vi "WILT Step 2.vi"(0 "Dryer Input":T4 {"Night Cycle Count" format="%04d"; "Day Cycle Count" format="%04d"}, 1 "Station Number in":u32, 3 "Send Restart Every? (Sec)":dbl=7.0 format="%#_13g", 5 "Station Test State Cluster":T2, 9 "Current Threshold":dbl=1.0 format="%#_13g", 11 "Error In":errorcluster, 12 "Enable Start Retry":bool, 13 "Delay After Cutout (sec)":dbl, 14 "Agilent Valve and Switch Locations":T1[](array[typedef])) -> (4 "Dryer Output":T4 {"Night Cycle Count" format="%04d"; "Day Cycle Count" format="%04d"}, 6 "Step 2 Output":T2, 10 "Resending Sending Command":bool, 15 "Error Out":errorcluster)   [LabVIEW 2016]
uses:
  Type Definitions/WILT Dryer.ctl
  Type Definitions/WILT Dryer Details.ctl
  Type Definitions/WILT Agilent Channel Definition.ctl
  Type Definitions/WILT DAQ Data.ctl
  Type Definitions/WILT Station Test State Cluster.ctl
  Type Definitions/WILT Dryer Test State.ctl
  Globals/WILT Globals Main Program.vi
panel:
  # "Day"
  # "Night"
  # "Day"
  # "Night"
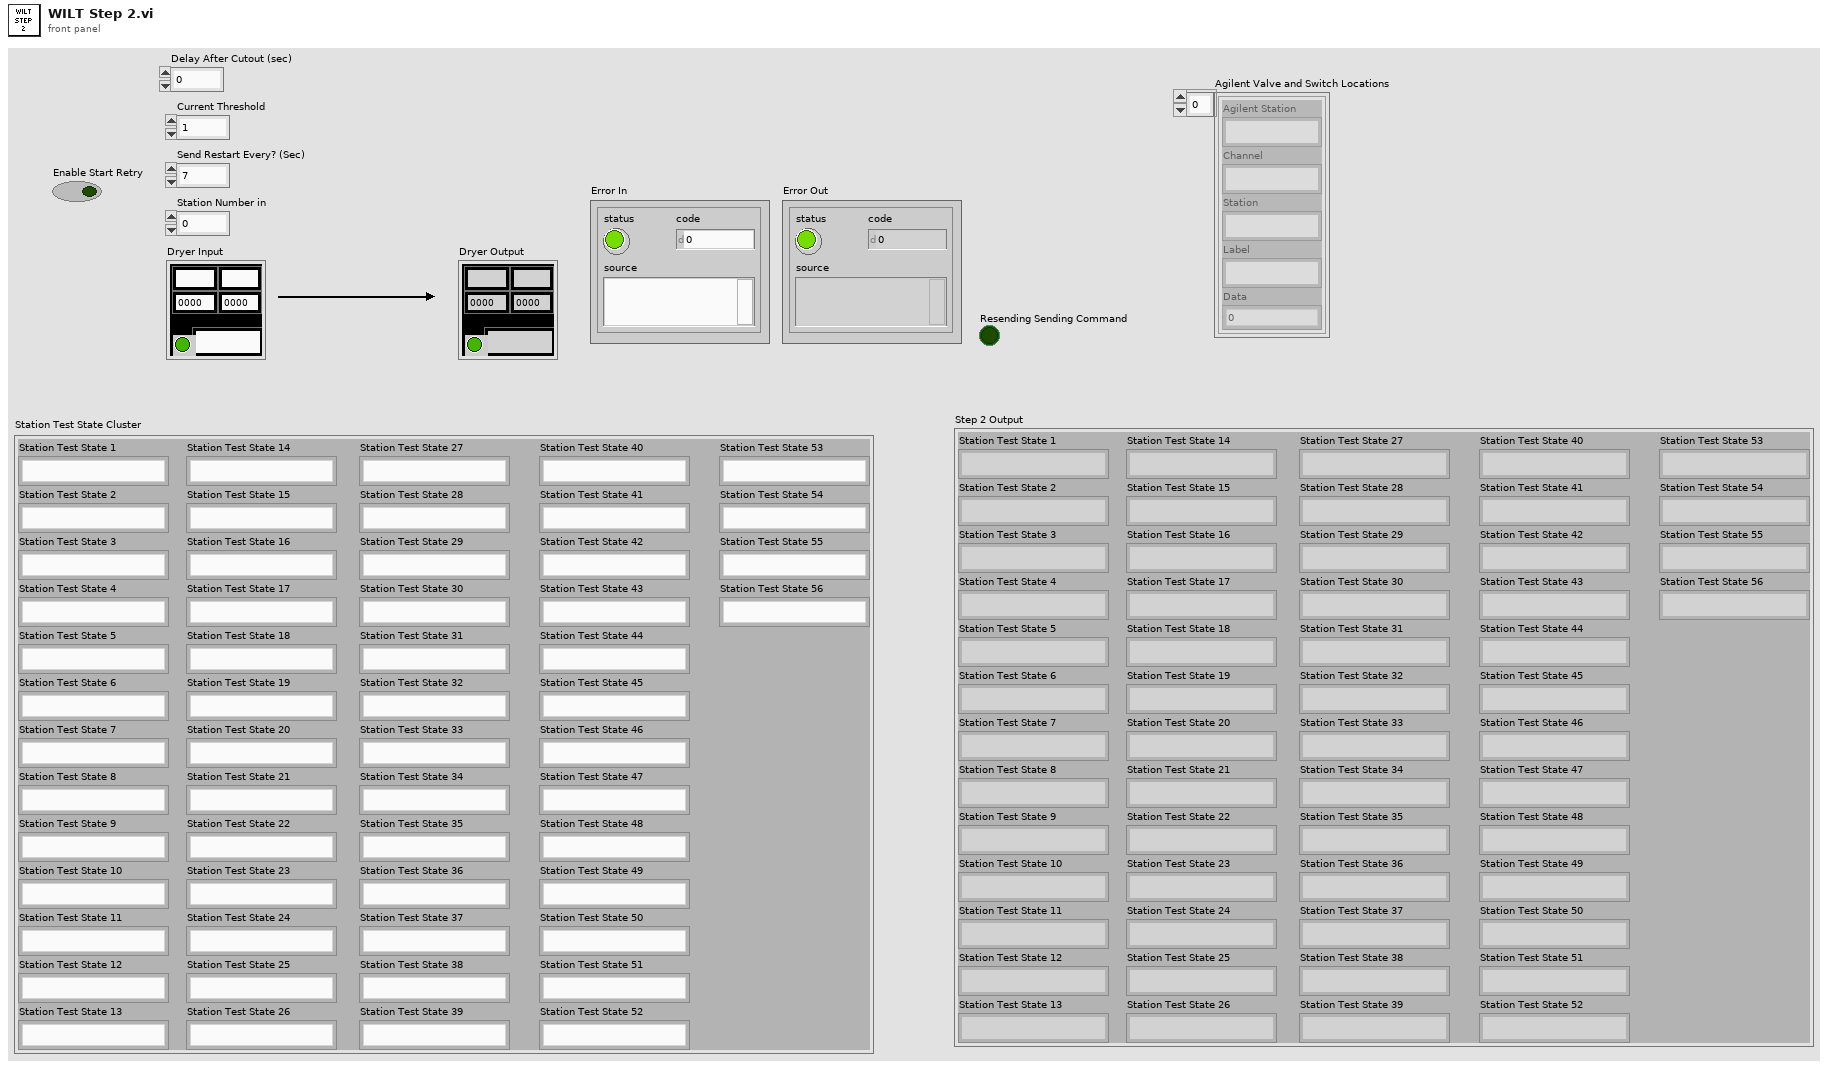
[diagram p1: front panel]
types:
  T1 = typedef "WILT Agilent Channel Definition.ctl" = cluster{"Channel":string, "Station":string, "Label":string, "Agilent Station":string, "Data":dbl}
  T2 = typedef "WILT Station Test State Cluster.ctl" = cluster{"Station Test State 1":T3, "Station Test State 2":T3, "Station Test State 3":T3, "Station Test State 4":T3, "Station Test State 5":T3, "Station Test State 6":T3, "Station Test State 7":T3, "Station Test State 8":T3, "Station Test State 9":T3, "Station Test State 10":T3, "Station Test State 11":T3, "Station Test State 12":T3, "Station Test State 13":T3, "Station Test State 14":T3, "Station Test State 15":T3, "Station Test State 16":T3, "Station Test State 17":T3, "Station Test State 18":T3, "Station Test State 19":T3, "Station Test State 20":T3, "Station Test State 21":T3, "Station Test State 22":T3, "Station Test State 23":T3, "Station Test State 24":T3, "Station Test State 25":T3, "Station Test State 26":T3, "Station Test State 27":T3, "Station Test State 28":T3, "Station Test State 29":T3, "Station Test State 30":T3, "Station Test State 31":T3, "Station Test State 32":T3, "Station Test State 33":T3, "Station Test State 34":T3, "Station Test State 35":T3, "Station Test State 36":T3, "Station Test State 37":T3, "Station Test State 38":T3, "Station Test State 39":T3, "Station Test State 40":T3, "Station Test State 41":T3, "Station Test State 42":T3, "Station Test State 43":T3, "Station Test State 44":T3, "Station Test State 45":T3, "Station Test State 46":T3, "Station Test State 47":T3, "Station Test State 48":T3, "Station Test State 49":T3, "Station Test State 50":T3, "Station Test State 51":T3, "Station Test State 52":T3, "Station Test State 53":T3, "Station Test State 54":T3, "Station Test State 55":T3, "Station Test State 56":T3}
  T3 = typedef "WILT Dryer Test State.ctl" = enum16{"No Serial Number", "Waiting for Dryer To Start", "Drying Clothes", "Water Injection 1 (On)", "Water Injection 1 Timer", "Water Injection 1 (Off)", "Pause Dryer", "Sending Start Stop CMD", "Pause Dryer 2", "Sending Start Stop CMD 2", "Drying Clothes 2", "Water Injection 2 (On)", "Water Injection 2 Timer", "Water Injection 2 (Off)", "Drying Clothes 3", "Cooling Down", "Sending Start Stop CMD 3", "Increment Cycle"}
  T4 = typedef "WILT Dryer.ctl" = cluster{"Lab ID":string, "Day Cycle Count":i32, "Station Label":string, "Dryer Details":T5, "Status Color":u32, "Invisible Button":bool, "Night Cycle Count":i32, "Station Index":i32, "Cycle Index":string, "Audit Alert":bool, "Agilent Channel Definition":T1, "DAQ Data":T6}
  T5 = typedef "WILT Dryer Details.ctl" = cluster{"Station":string, "Lab ID":string, "TR Number":string}
  T6 = typedef "WILT DAQ Data.ctl" = cluster{"L1 Current":dbl, "L2 Current":dbl, "Temperature  Deg F (TC)":dbl, "Volts":dbl, "Volts (208)":dbl, "SW (208)":dbl}
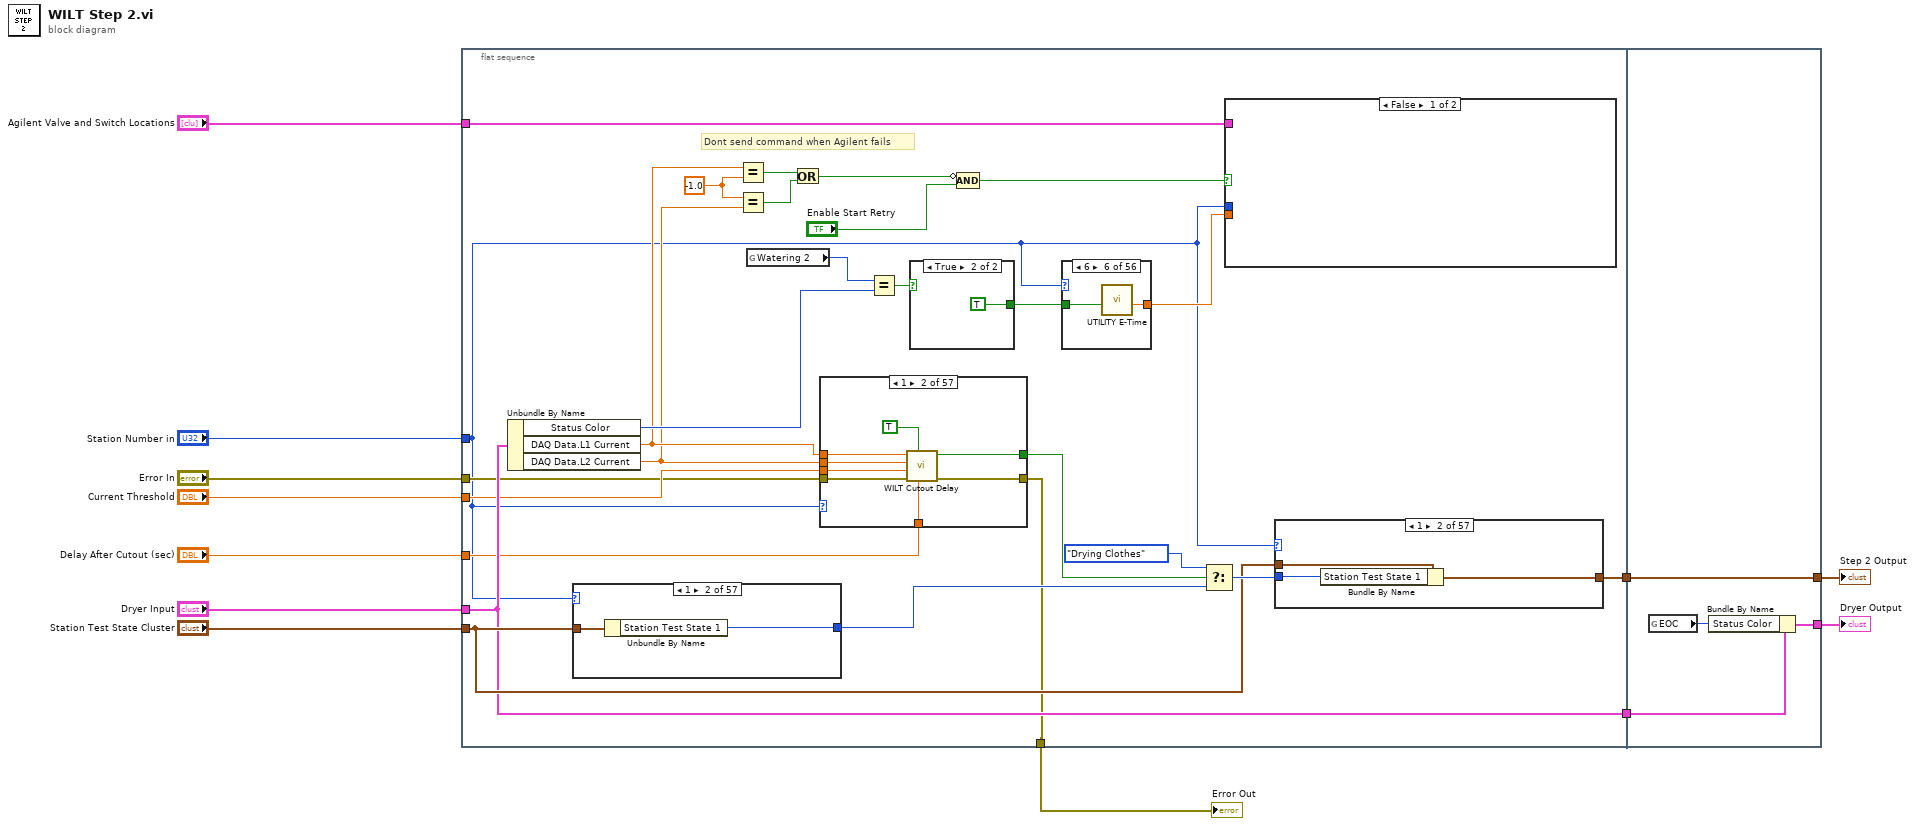
[diagram p0: block diagram]
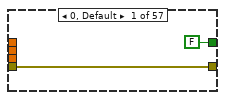
[diagram p2: hidden frame]
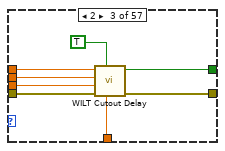
[diagram p3: hidden frame]
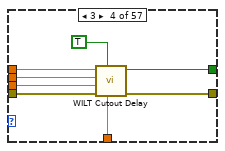
[diagram p4: hidden frame]
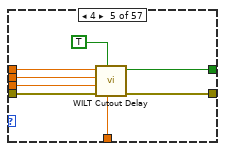
[diagram p5: hidden frame]
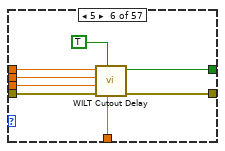
[diagram p6: hidden frame]
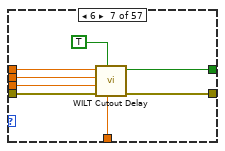
[diagram p7: hidden frame]
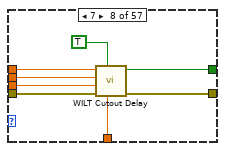
[diagram p8: hidden frame]
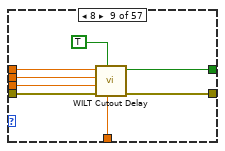
[diagram p9: hidden frame]
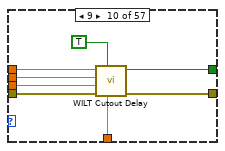
[diagram p10: hidden frame]
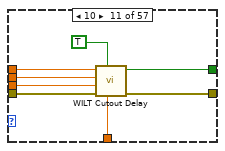
[diagram p11: hidden frame]
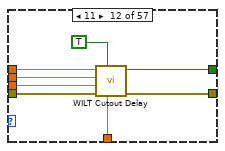
[diagram p12: hidden frame]
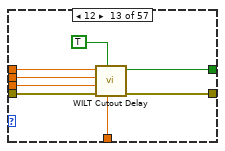
[diagram p13: hidden frame]
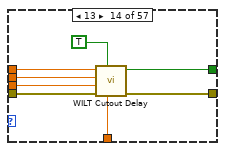
[diagram p14: hidden frame]
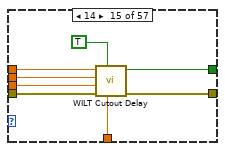
[diagram p15: hidden frame]
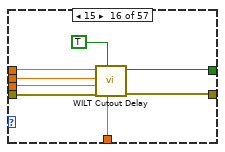
[diagram p16: hidden frame]
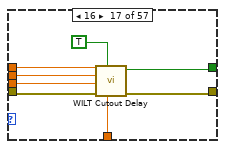
[diagram p17: hidden frame]
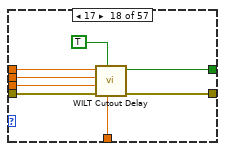
[diagram p18: hidden frame]
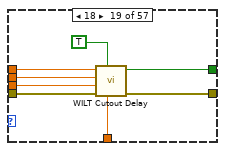
[diagram p19: hidden frame]
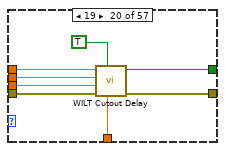
[diagram p20: hidden frame]
diagram:
  n1 = flat-sequence {
    tunnel: "Current Threshold" -> [w18]
    tunnel: "Station Test State Cluster" -> [w35]
    tunnel: "Station Number in" -> [w13]
    tunnel: [w38] -> w8
    tunnel: "Dryer Input" -> [w29]
    tunnel: [w29] -> w6
    tunnel: "Agilent Valve and Switch Locations" -> [w27]
    tunnel: [w16] -> w3
    tunnel: "Error In" -> [w15]
    tunnel: "Delay After Cutout (sec)" -> [w14]
    tunnel: [w893] -> w12
    tunnel: w8 -> [w893]
    tunnel: [w891] -> w7
    tunnel: w6 -> [w890]
    frame #0 {
      w26 = -1.0 ("x")
      # "Dont send command when Agilent fails"
      n2 = Unbundle By Name(w29) -> ("Status Color"=w33:u32, "DAQ Data.L1 Current"=w20:dbl, "DAQ Data.L2 Current"=w19:dbl)
      n3 = case shown="1" w13 {
        tunnel: w35 -> [_ w610 w612 w614 w616 w618 w620 w622 w624 w626 w628 w630 w632 w634 w636 w638 w640 w642 w644 w646 w648 w650 w652 w654 w656 w658 w660 w662 w664 w666 w668 w670 w672 w674 w676 w678 w680 w682 w684 w686 w688 w690 w692 w694 w696 w698 w700 w702 w704 w706 w708 w710 w712 w714 w716 w718 w720]
        tunnel: [WILT_Dryer_Test_State."No Serial Number" ("Station Test State 56") w609 w611 w613 w615 w617 w619 w621 w623 w625 w627 w629 w631 w633 w635 w637 w639 w641 w643 w645 w647 w649 w651 w653 w655 w657 w659 w661 w663 w665 w667 w669 w671 w673 w675 w677 w679 w681 w683 w685 w687 w689 w691 w693 w695 w697 w699 w701 w703 w705 w707 w709 w711 w713 w715 w717 w719] -> w34
        frame 0, Default {
          # "This is not a station.\nDo nothing"
        }
        frame 1 {
          n4 = Unbundle By Name(w610) -> ("Station Test State 1"=w609:T3)
        }
        frame 2 {
          n5 = Unbundle By Name(w612) -> ("Station Test State 2"=w611:T3)
        }
        frame 3 {
          n6 = Unbundle By Name(w614) -> ("Station Test State 3"=w613:T3)
        }
        frame 4 {
          n7 = Unbundle By Name(w616) -> ("Station Test State 4"=w615:T3)
        }
        frame 5 {
          n8 = Unbundle By Name(w618) -> ("Station Test State 5"=w617:T3)
        }
        frame 6 {
          n9 = Unbundle By Name(w620) -> ("Station Test State 6"=w619:T3)
        }
        frame 7 {
          n10 = Unbundle By Name(w622) -> ("Station Test State 7"=w621:T3)
        }
        frame 8 {
          n11 = Unbundle By Name(w624) -> ("Station Test State 8"=w623:T3)
        }
        frame 9 {
          n12 = Unbundle By Name(w626) -> ("Station Test State 9"=w625:T3)
        }
        frame 10 {
          n13 = Unbundle By Name(w628) -> ("Station Test State 10"=w627:T3)
        }
        frame 11 {
          n14 = Unbundle By Name(w630) -> ("Station Test State 11"=w629:T3)
        }
        frame 12 {
          n15 = Unbundle By Name(w632) -> ("Station Test State 12"=w631:T3)
        }
        frame 13 {
          n16 = Unbundle By Name(w634) -> ("Station Test State 13"=w633:T3)
        }
        frame 14 {
          n17 = Unbundle By Name(w636) -> ("Station Test State 14"=w635:T3)
        }
        frame 15 {
          n18 = Unbundle By Name(w638) -> ("Station Test State 15"=w637:T3)
        }
        frame 16 {
          n19 = Unbundle By Name(w640) -> ("Station Test State 16"=w639:T3)
        }
        frame 17 {
          n20 = Unbundle By Name(w642) -> ("Station Test State 17"=w641:T3)
        }
        frame 18 {
          n21 = Unbundle By Name(w644) -> ("Station Test State 18"=w643:T3)
        }
        frame 19 {
          n22 = Unbundle By Name(w646) -> ("Station Test State 19"=w645:T3)
        }
        frame 20 {
          n23 = Unbundle By Name(w648) -> ("Station Test State 20"=w647:T3)
        }
        frame 21 {
          n24 = Unbundle By Name(w650) -> ("Station Test State 21"=w649:T3)
        }
        frame 22 {
          n25 = Unbundle By Name(w652) -> ("Station Test State 22"=w651:T3)
        }
        frame 23 {
          n26 = Unbundle By Name(w654) -> ("Station Test State 23"=w653:T3)
        }
        frame 24 {
          n27 = Unbundle By Name(w656) -> ("Station Test State 24"=w655:T3)
        }
        frame 25 {
          n28 = Unbundle By Name(w658) -> ("Station Test State 25"=w657:T3)
        }
        frame 26 {
          n29 = Unbundle By Name(w660) -> ("Station Test State 26"=w659:T3)
        }
        frame 27 {
          n30 = Unbundle By Name(w662) -> ("Station Test State 27"=w661:T3)
        }
        frame 28 {
          n31 = Unbundle By Name(w664) -> ("Station Test State 28"=w663:T3)
        }
        frame 29 {
          n32 = Unbundle By Name(w666) -> ("Station Test State 29"=w665:T3)
        }
        frame 30 {
          n33 = Unbundle By Name(w668) -> ("Station Test State 30"=w667:T3)
        }
        frame 31 {
          n34 = Unbundle By Name(w670) -> ("Station Test State 31"=w669:T3)
        }
        frame 32 {
          n35 = Unbundle By Name(w672) -> ("Station Test State 32"=w671:T3)
        }
        frame 33 {
          n36 = Unbundle By Name(w674) -> ("Station Test State 33"=w673:T3)
        }
        frame 34 {
          n37 = Unbundle By Name(w676) -> ("Station Test State 34"=w675:T3)
        }
        frame 35 {
          n38 = Unbundle By Name(w678) -> ("Station Test State 35"=w677:T3)
        }
        frame 36 {
          n39 = Unbundle By Name(w680) -> ("Station Test State 36"=w679:T3)
        }
        frame 37 {
          n40 = Unbundle By Name(w682) -> ("Station Test State 37"=w681:T3)
        }
        frame 38 {
          n41 = Unbundle By Name(w684) -> ("Station Test State 38"=w683:T3)
        }
        frame 39 {
          n42 = Unbundle By Name(w686) -> ("Station Test State 39"=w685:T3)
        }
        frame 40 {
          n43 = Unbundle By Name(w688) -> ("Station Test State 40"=w687:T3)
        }
        frame 41 {
          n44 = Unbundle By Name(w690) -> ("Station Test State 41"=w689:T3)
        }
        frame 42 {
          n45 = Unbundle By Name(w692) -> ("Station Test State 42"=w691:T3)
        }
        frame 43 {
          n46 = Unbundle By Name(w694) -> ("Station Test State 43"=w693:T3)
        }
        frame 44 {
          n47 = Unbundle By Name(w696) -> ("Station Test State 44"=w695:T3)
        }
        frame 45 {
          n48 = Unbundle By Name(w698) -> ("Station Test State 45"=w697:T3)
        }
        frame 46 {
          n49 = Unbundle By Name(w700) -> ("Station Test State 46"=w699:T3)
        }
        frame 47 {
          n50 = Unbundle By Name(w702) -> ("Station Test State 47"=w701:T3)
        }
        frame 48 {
          n51 = Unbundle By Name(w704) -> ("Station Test State 48"=w703:T3)
        }
        frame 49 {
          n52 = Unbundle By Name(w706) -> ("Station Test State 49"=w705:T3)
        }
        frame 50 {
          n53 = Unbundle By Name(w708) -> ("Station Test State 50"=w707:T3)
        }
        frame 51 {
          n54 = Unbundle By Name(w710) -> ("Station Test State 51"=w709:T3)
        }
        frame 52 {
          n55 = Unbundle By Name(w712) -> ("Station Test State 52"=w711:T3)
        }
        frame 53 {
          n56 = Unbundle By Name(w714) -> ("Station Test State 53"=w713:T3)
        }
        frame 54 {
          n57 = Unbundle By Name(w716) -> ("Station Test State 54"=w715:T3)
        }
        frame 55 {
          n58 = Unbundle By Name(w718) -> ("Station Test State 55"=w717:T3)
        }
        frame 56 {
          n59 = Unbundle By Name(w720) -> ("Station Test State 56"=w719:T3)
        }
      }
      n60 = Equal?(x=w20, y=w26) -> (x = y?=w25:bool)
      n61 = Equal?(x=w26, y=w19) -> (x = y?=w24:bool)
      n62 = global read "WILT Globals Main Program.vi" "Watering 2"() -> (w32:u32)
      n63 = Or(x=w25, y=w24) -> (x .or. y?=w22:bool)
      n64 = case shown="1" w13 {
        tunnel: w18 -> [_ w48 w51 w59 w70 w78 w86 w94 w102 w110 w118 w126 w134 w142 w150 w155 w166 w174 w182 w190 w198 w206 w214 w222 w230 w238 w246 w254 w262 w270 w278 w286 w294 w302 w310 w318 w326 w334 w342 w350 w358 w366 w374 w382 w390 w398 w406 w414 w422 w430 w438 w446 w454 w462 w470 w478 w486]
        tunnel: w20 -> [_ w47 w53 w61 w72 w80 w88 w96 w104 w112 w120 w128 w136 w144 w152 w157 w168 w176 w184 w192 w200 w208 w216 w224 w232 w240 w248 w256 w264 w272 w280 w288 w296 w304 w312 w320 w328 w336 w344 w352 w360 w368 w376 w384 w392 w400 w408 w416 w424 w432 w440 w448 w456 w464 w472 w480 w488]
        tunnel: w19 -> [_ w46 w52 w60 w71 w79 w87 w95 w103 w111 w119 w127 w135 w143 w151 w156 w167 w175 w183 w191 w199 w207 w215 w223 w231 w239 w247 w255 w263 w271 w279 w287 w295 w303 w311 w319 w327 w335 w343 w351 w359 w367 w375 w383 w391 w399 w407 w415 w423 w431 w439 w447 w455 w463 w471 w479 w487]
        tunnel: [FALSE ("Delayed Trigger") w45 w50 w62 w66 w75 w83 w90 w99 w107 w115 w122 w132 w140 w148 w158 w163 w171 w179 w188 w195 w202 w211 w218 w227 w235 w242 w251 w259 w267 w275 w282 w290 w298 w306 w314 w323 w330 w338 w347 w354 w362 w370 w378 w387 w395 w402 w411 w418 w427 w435 w443 w451 w459 w467 w475 w482] -> w17
        tunnel: w15 -> [w40 w44 w56 w64 w69 w77 w85 w93 w101 w109 w117 w125 w133 w141 w149 w160 w165 w173 w181 w189 w197 w205 w213 w221 w229 w237 w245 w253 w261 w269 w277 w285 w293 w301 w309 w317 w325 w333 w341 w349 w357 w365 w373 w381 w389 w397 w405 w413 w421 w429 w437 w445 w453 w461 w469 w477 w485]
        tunnel: [w40 w43 w55 w63 w67 w76 w82 w91 w100 w108 w114 w123 w131 w139 w147 w159 w164 w172 w180 w187 w196 w203 w210 w219 w228 w234 w243 w252 w260 w268 w276 w283 w291 w299 w307 w315 w324 w331 w339 w348 w355 w363 w371 w379 w388 w396 w403 w412 w419 w428 w436 w444 w452 w460 w468 w476 w483] -> w16
        tunnel: w14 -> [_ w42 w54 w58 w68 w74 w84 w92 w98 w106 w116 w124 w130 w138 w146 w154 w162 w170 w178 w186 w194 w204 w212 w220 w226 w236 w244 w250 w258 w266 w274 w284 w292 w300 w308 w316 w322 w332 w340 w346 w356 w364 w372 w380 w386 w394 w404 w410 w420 w426 w434 w442 w450 w458 w466 w474 w484]
        frame 0, Default {
        }
        frame 1 {
          n65 = call "WILT Cutout Delay.vi"("Delay After Cutout (sec)"=w42, "Cut-In?"=TRUE, "Error In"=w44, "Current Threshold"=w48, "L2 Current"=w46, "L1 Current"=w47) -> ("Error Out"=w43:errorcluster, "Delayed Trigger"=w45:bool)  [unwired: 2 in, 2 out]
        }
        frame 2 {
          n66 = call "WILT Cutout Delay.vi"("Delay After Cutout (sec)"=w54, "Cut-In?"=TRUE, "Error In"=w56, "Current Threshold"=w51, "L2 Current"=w52, "L1 Current"=w53) -> ("Error Out"=w55:errorcluster, "Delayed Trigger"=w50:bool)  [unwired: 2 in, 2 out]
        }
        frame 3 {
          n67 = call "WILT Cutout Delay.vi"("Delay After Cutout (sec)"=w58, "Cut-In?"=TRUE, "Error In"=w64, "Current Threshold"=w59, "L2 Current"=w60, "L1 Current"=w61) -> ("Error Out"=w63:errorcluster, "Delayed Trigger"=w62:bool)  [unwired: 2 in, 2 out]
        }
        frame 4 {
          n68 = call "WILT Cutout Delay.vi"("Delay After Cutout (sec)"=w68, "Cut-In?"=TRUE, "Error In"=w69, "Current Threshold"=w70, "L2 Current"=w71, "L1 Current"=w72) -> ("Error Out"=w67:errorcluster, "Delayed Trigger"=w66:bool)  [unwired: 2 in, 2 out]
        }
        frame 5 {
          n69 = call "WILT Cutout Delay.vi"("Delay After Cutout (sec)"=w74, "Cut-In?"=TRUE, "Error In"=w77, "Current Threshold"=w78, "L2 Current"=w79, "L1 Current"=w80) -> ("Error Out"=w76:errorcluster, "Delayed Trigger"=w75:bool)  [unwired: 2 in, 2 out]
        }
        frame 6 {
          n70 = call "WILT Cutout Delay.vi"("Delay After Cutout (sec)"=w84, "Cut-In?"=TRUE, "Error In"=w85, "Current Threshold"=w86, "L2 Current"=w87, "L1 Current"=w88) -> ("Error Out"=w82:errorcluster, "Delayed Trigger"=w83:bool)  [unwired: 2 in, 2 out]
        }
        frame 7 {
          n71 = call "WILT Cutout Delay.vi"("Delay After Cutout (sec)"=w92, "Cut-In?"=TRUE, "Error In"=w93, "Current Threshold"=w94, "L2 Current"=w95, "L1 Current"=w96) -> ("Error Out"=w91:errorcluster, "Delayed Trigger"=w90:bool)  [unwired: 2 in, 2 out]
        }
        frame 8 {
          n72 = call "WILT Cutout Delay.vi"("Delay After Cutout (sec)"=w98, "Cut-In?"=TRUE, "Error In"=w101, "Current Threshold"=w102, "L2 Current"=w103, "L1 Current"=w104) -> ("Error Out"=w100:errorcluster, "Delayed Trigger"=w99:bool)  [unwired: 2 in, 2 out]
        }
        frame 9 {
          n73 = call "WILT Cutout Delay.vi"("Delay After Cutout (sec)"=w106, "Cut-In?"=TRUE, "Error In"=w109, "Current Threshold"=w110, "L2 Current"=w111, "L1 Current"=w112) -> ("Error Out"=w108:errorcluster, "Delayed Trigger"=w107:bool)  [unwired: 2 in, 2 out]
        }
        frame 10 {
          n74 = call "WILT Cutout Delay.vi"("Delay After Cutout (sec)"=w116, "Cut-In?"=TRUE, "Error In"=w117, "Current Threshold"=w118, "L2 Current"=w119, "L1 Current"=w120) -> ("Error Out"=w114:errorcluster, "Delayed Trigger"=w115:bool)  [unwired: 2 in, 2 out]
        }
        frame 11 {
          n75 = call "WILT Cutout Delay.vi"("Delay After Cutout (sec)"=w124, "Cut-In?"=TRUE, "Error In"=w125, "Current Threshold"=w126, "L2 Current"=w127, "L1 Current"=w128) -> ("Error Out"=w123:errorcluster, "Delayed Trigger"=w122:bool)  [unwired: 2 in, 2 out]
        }
        frame 12 {
          n76 = call "WILT Cutout Delay.vi"("Delay After Cutout (sec)"=w130, "Cut-In?"=TRUE, "Error In"=w133, "Current Threshold"=w134, "L2 Current"=w135, "L1 Current"=w136) -> ("Error Out"=w131:errorcluster, "Delayed Trigger"=w132:bool)  [unwired: 2 in, 2 out]
        }
        frame 13 {
          n77 = call "WILT Cutout Delay.vi"("Delay After Cutout (sec)"=w138, "Cut-In?"=TRUE, "Error In"=w141, "Current Threshold"=w142, "L2 Current"=w143, "L1 Current"=w144) -> ("Error Out"=w139:errorcluster, "Delayed Trigger"=w140:bool)  [unwired: 2 in, 2 out]
        }
        frame 14 {
          n78 = call "WILT Cutout Delay.vi"("Delay After Cutout (sec)"=w146, "Cut-In?"=TRUE, "Error In"=w149, "Current Threshold"=w150, "L2 Current"=w151, "L1 Current"=w152) -> ("Error Out"=w147:errorcluster, "Delayed Trigger"=w148:bool)  [unwired: 2 in, 2 out]
        }
        frame 15 {
          n79 = call "WILT Cutout Delay.vi"("Delay After Cutout (sec)"=w154, "Cut-In?"=TRUE, "Error In"=w160, "Current Threshold"=w155, "L2 Current"=w156, "L1 Current"=w157) -> ("Error Out"=w159:errorcluster, "Delayed Trigger"=w158:bool)  [unwired: 2 in, 2 out]
        }
        frame 16 {
          n80 = call "WILT Cutout Delay.vi"("Delay After Cutout (sec)"=w162, "Cut-In?"=TRUE, "Error In"=w165, "Current Threshold"=w166, "L2 Current"=w167, "L1 Current"=w168) -> ("Error Out"=w164:errorcluster, "Delayed Trigger"=w163:bool)  [unwired: 2 in, 2 out]
        }
        frame 17 {
          n81 = call "WILT Cutout Delay.vi"("Delay After Cutout (sec)"=w170, "Cut-In?"=TRUE, "Error In"=w173, "Current Threshold"=w174, "L2 Current"=w175, "L1 Current"=w176) -> ("Error Out"=w172:errorcluster, "Delayed Trigger"=w171:bool)  [unwired: 2 in, 2 out]
        }
        frame 18 {
          n82 = call "WILT Cutout Delay.vi"("Delay After Cutout (sec)"=w178, "Cut-In?"=TRUE, "Error In"=w181, "Current Threshold"=w182, "L2 Current"=w183, "L1 Current"=w184) -> ("Error Out"=w180:errorcluster, "Delayed Trigger"=w179:bool)  [unwired: 2 in, 2 out]
        }
        frame 19 {
          n83 = call "WILT Cutout Delay.vi"("Delay After Cutout (sec)"=w186, "Cut-In?"=TRUE, "Error In"=w189, "Current Threshold"=w190, "L2 Current"=w191, "L1 Current"=w192) -> ("Error Out"=w187:errorcluster, "Delayed Trigger"=w188:bool)  [unwired: 2 in, 2 out]
        }
        frame 20 {
          n84 = call "WILT Cutout Delay.vi"("Delay After Cutout (sec)"=w194, "Cut-In?"=TRUE, "Error In"=w197, "Current Threshold"=w198, "L2 Current"=w199, "L1 Current"=w200) -> ("Error Out"=w196:errorcluster, "Delayed Trigger"=w195:bool)  [unwired: 2 in, 2 out]
        }
        frame 21 {
          n85 = call "WILT Cutout Delay.vi"("Delay After Cutout (sec)"=w204, "Cut-In?"=TRUE, "Error In"=w205, "Current Threshold"=w206, "L2 Current"=w207, "L1 Current"=w208) -> ("Error Out"=w203:errorcluster, "Delayed Trigger"=w202:bool)  [unwired: 2 in, 2 out]
        }
        frame 22 {
          n86 = call "WILT Cutout Delay.vi"("Delay After Cutout (sec)"=w212, "Cut-In?"=TRUE, "Error In"=w213, "Current Threshold"=w214, "L2 Current"=w215, "L1 Current"=w216) -> ("Error Out"=w210:errorcluster, "Delayed Trigger"=w211:bool)  [unwired: 2 in, 2 out]
        }
        frame 23 {
          n87 = call "WILT Cutout Delay.vi"("Delay After Cutout (sec)"=w220, "Cut-In?"=TRUE, "Error In"=w221, "Current Threshold"=w222, "L2 Current"=w223, "L1 Current"=w224) -> ("Error Out"=w219:errorcluster, "Delayed Trigger"=w218:bool)  [unwired: 2 in, 2 out]
        }
        frame 24 {
          n88 = call "WILT Cutout Delay.vi"("Delay After Cutout (sec)"=w226, "Cut-In?"=TRUE, "Error In"=w229, "Current Threshold"=w230, "L2 Current"=w231, "L1 Current"=w232) -> ("Error Out"=w228:errorcluster, "Delayed Trigger"=w227:bool)  [unwired: 2 in, 2 out]
        }
        frame 25 {
          n89 = call "WILT Cutout Delay.vi"("Delay After Cutout (sec)"=w236, "Cut-In?"=TRUE, "Error In"=w237, "Current Threshold"=w238, "L2 Current"=w239, "L1 Current"=w240) -> ("Error Out"=w234:errorcluster, "Delayed Trigger"=w235:bool)  [unwired: 2 in, 2 out]
        }
        frame 26 {
          n90 = call "WILT Cutout Delay.vi"("Delay After Cutout (sec)"=w244, "Cut-In?"=TRUE, "Error In"=w245, "Current Threshold"=w246, "L2 Current"=w247, "L1 Current"=w248) -> ("Error Out"=w243:errorcluster, "Delayed Trigger"=w242:bool)  [unwired: 2 in, 2 out]
        }
        frame 27 {
          n91 = call "WILT Cutout Delay.vi"("Delay After Cutout (sec)"=w250, "Cut-In?"=TRUE, "Error In"=w253, "Current Threshold"=w254, "L2 Current"=w255, "L1 Current"=w256) -> ("Error Out"=w252:errorcluster, "Delayed Trigger"=w251:bool)  [unwired: 2 in, 2 out]
        }
        frame 28 {
          n92 = call "WILT Cutout Delay.vi"("Delay After Cutout (sec)"=w258, "Cut-In?"=TRUE, "Error In"=w261, "Current Threshold"=w262, "L2 Current"=w263, "L1 Current"=w264) -> ("Error Out"=w260:errorcluster, "Delayed Trigger"=w259:bool)  [unwired: 2 in, 2 out]
        }
        frame 29 {
          n93 = call "WILT Cutout Delay.vi"("Delay After Cutout (sec)"=w266, "Cut-In?"=TRUE, "Error In"=w269, "Current Threshold"=w270, "L2 Current"=w271, "L1 Current"=w272) -> ("Error Out"=w268:errorcluster, "Delayed Trigger"=w267:bool)  [unwired: 2 in, 2 out]
        }
        frame 30 {
          n94 = call "WILT Cutout Delay.vi"("Delay After Cutout (sec)"=w274, "Cut-In?"=TRUE, "Error In"=w277, "Current Threshold"=w278, "L2 Current"=w279, "L1 Current"=w280) -> ("Error Out"=w276:errorcluster, "Delayed Trigger"=w275:bool)  [unwired: 2 in, 2 out]
        }
        frame 31 {
          n95 = call "WILT Cutout Delay.vi"("Delay After Cutout (sec)"=w284, "Cut-In?"=TRUE, "Error In"=w285, "Current Threshold"=w286, "L2 Current"=w287, "L1 Current"=w288) -> ("Error Out"=w283:errorcluster, "Delayed Trigger"=w282:bool)  [unwired: 2 in, 2 out]
        }
        frame 32 {
          n96 = call "WILT Cutout Delay.vi"("Delay After Cutout (sec)"=w292, "Cut-In?"=TRUE, "Error In"=w293, "Current Threshold"=w294, "L2 Current"=w295, "L1 Current"=w296) -> ("Error Out"=w291:errorcluster, "Delayed Trigger"=w290:bool)  [unwired: 2 in, 2 out]
        }
        frame 33 {
          n97 = call "WILT Cutout Delay.vi"("Delay After Cutout (sec)"=w300, "Cut-In?"=TRUE, "Error In"=w301, "Current Threshold"=w302, "L2 Current"=w303, "L1 Current"=w304) -> ("Error Out"=w299:errorcluster, "Delayed Trigger"=w298:bool)  [unwired: 2 in, 2 out]
        }
        frame 34 {
          n98 = call "WILT Cutout Delay.vi"("Delay After Cutout (sec)"=w308, "Cut-In?"=TRUE, "Error In"=w309, "Current Threshold"=w310, "L2 Current"=w311, "L1 Current"=w312) -> ("Error Out"=w307:errorcluster, "Delayed Trigger"=w306:bool)  [unwired: 2 in, 2 out]
        }
        frame 35 {
          n99 = call "WILT Cutout Delay.vi"("Delay After Cutout (sec)"=w316, "Cut-In?"=TRUE, "Error In"=w317, "Current Threshold"=w318, "L2 Current"=w319, "L1 Current"=w320) -> ("Error Out"=w315:errorcluster, "Delayed Trigger"=w314:bool)  [unwired: 2 in, 2 out]
        }
        frame 36 {
          n100 = call "WILT Cutout Delay.vi"("Delay After Cutout (sec)"=w322, "Cut-In?"=TRUE, "Error In"=w325, "Current Threshold"=w326, "L2 Current"=w327, "L1 Current"=w328) -> ("Error Out"=w324:errorcluster, "Delayed Trigger"=w323:bool)  [unwired: 2 in, 2 out]
        }
        frame 37 {
          n101 = call "WILT Cutout Delay.vi"("Delay After Cutout (sec)"=w332, "Cut-In?"=TRUE, "Error In"=w333, "Current Threshold"=w334, "L2 Current"=w335, "L1 Current"=w336) -> ("Error Out"=w331:errorcluster, "Delayed Trigger"=w330:bool)  [unwired: 2 in, 2 out]
        }
        frame 38 {
          n102 = call "WILT Cutout Delay.vi"("Delay After Cutout (sec)"=w340, "Cut-In?"=TRUE, "Error In"=w341, "Current Threshold"=w342, "L2 Current"=w343, "L1 Current"=w344) -> ("Error Out"=w339:errorcluster, "Delayed Trigger"=w338:bool)  [unwired: 2 in, 2 out]
        }
        frame 39 {
          n103 = call "WILT Cutout Delay.vi"("Delay After Cutout (sec)"=w346, "Cut-In?"=TRUE, "Error In"=w349, "Current Threshold"=w350, "L2 Current"=w351, "L1 Current"=w352) -> ("Error Out"=w348:errorcluster, "Delayed Trigger"=w347:bool)  [unwired: 2 in, 2 out]
        }
        frame 40 {
          n104 = call "WILT Cutout Delay.vi"("Delay After Cutout (sec)"=w356, "Cut-In?"=TRUE, "Error In"=w357, "Current Threshold"=w358, "L2 Current"=w359, "L1 Current"=w360) -> ("Error Out"=w355:errorcluster, "Delayed Trigger"=w354:bool)  [unwired: 2 in, 2 out]
        }
        frame 41 {
          n105 = call "WILT Cutout Delay.vi"("Delay After Cutout (sec)"=w364, "Cut-In?"=TRUE, "Error In"=w365, "Current Threshold"=w366, "L2 Current"=w367, "L1 Current"=w368) -> ("Error Out"=w363:errorcluster, "Delayed Trigger"=w362:bool)  [unwired: 2 in, 2 out]
        }
        frame 42 {
          n106 = call "WILT Cutout Delay.vi"("Delay After Cutout (sec)"=w372, "Cut-In?"=TRUE, "Error In"=w373, "Current Threshold"=w374, "L2 Current"=w375, "L1 Current"=w376) -> ("Error Out"=w371:errorcluster, "Delayed Trigger"=w370:bool)  [unwired: 2 in, 2 out]
        }
        frame 43 {
          n107 = call "WILT Cutout Delay.vi"("Delay After Cutout (sec)"=w380, "Cut-In?"=TRUE, "Error In"=w381, "Current Threshold"=w382, "L2 Current"=w383, "L1 Current"=w384) -> ("Error Out"=w379:errorcluster, "Delayed Trigger"=w378:bool)  [unwired: 2 in, 2 out]
        }
        frame 44 {
          n108 = call "WILT Cutout Delay.vi"("Delay After Cutout (sec)"=w386, "Cut-In?"=TRUE, "Error In"=w389, "Current Threshold"=w390, "L2 Current"=w391, "L1 Current"=w392) -> ("Error Out"=w388:errorcluster, "Delayed Trigger"=w387:bool)  [unwired: 2 in, 2 out]
        }
        frame 45 {
          n109 = call "WILT Cutout Delay.vi"("Delay After Cutout (sec)"=w394, "Cut-In?"=TRUE, "Error In"=w397, "Current Threshold"=w398, "L2 Current"=w399, "L1 Current"=w400) -> ("Error Out"=w396:errorcluster, "Delayed Trigger"=w395:bool)  [unwired: 2 in, 2 out]
        }
        frame 46 {
          n110 = call "WILT Cutout Delay.vi"("Delay After Cutout (sec)"=w404, "Cut-In?"=TRUE, "Error In"=w405, "Current Threshold"=w406, "L2 Current"=w407, "L1 Current"=w408) -> ("Error Out"=w403:errorcluster, "Delayed Trigger"=w402:bool)  [unwired: 2 in, 2 out]
        }
        frame 47 {
          n111 = call "WILT Cutout Delay.vi"("Delay After Cutout (sec)"=w410, "Cut-In?"=TRUE, "Error In"=w413, "Current Threshold"=w414, "L2 Current"=w415, "L1 Current"=w416) -> ("Error Out"=w412:errorcluster, "Delayed Trigger"=w411:bool)  [unwired: 2 in, 2 out]
        }
        frame 48 {
          n112 = call "WILT Cutout Delay.vi"("Delay After Cutout (sec)"=w420, "Cut-In?"=TRUE, "Error In"=w421, "Current Threshold"=w422, "L2 Current"=w423, "L1 Current"=w424) -> ("Error Out"=w419:errorcluster, "Delayed Trigger"=w418:bool)  [unwired: 2 in, 2 out]
        }
        frame 49 {
          n113 = call "WILT Cutout Delay.vi"("Delay After Cutout (sec)"=w426, "Cut-In?"=TRUE, "Error In"=w429, "Current Threshold"=w430, "L2 Current"=w431, "L1 Current"=w432) -> ("Error Out"=w428:errorcluster, "Delayed Trigger"=w427:bool)  [unwired: 2 in, 2 out]
        }
        frame 50 {
          n114 = call "WILT Cutout Delay.vi"("Delay After Cutout (sec)"=w434, "Cut-In?"=TRUE, "Error In"=w437, "Current Threshold"=w438, "L2 Current"=w439, "L1 Current"=w440) -> ("Error Out"=w436:errorcluster, "Delayed Trigger"=w435:bool)  [unwired: 2 in, 2 out]
        }
        frame 51 {
          n115 = call "WILT Cutout Delay.vi"("Delay After Cutout (sec)"=w442, "Cut-In?"=TRUE, "Error In"=w445, "Current Threshold"=w446, "L2 Current"=w447, "L1 Current"=w448) -> ("Error Out"=w444:errorcluster, "Delayed Trigger"=w443:bool)  [unwired: 2 in, 2 out]
        }
        frame 52 {
          n116 = call "WILT Cutout Delay.vi"("Delay After Cutout (sec)"=w450, "Cut-In?"=TRUE, "Error In"=w453, "Current Threshold"=w454, "L2 Current"=w455, "L1 Current"=w456) -> ("Error Out"=w452:errorcluster, "Delayed Trigger"=w451:bool)  [unwired: 2 in, 2 out]
        }
        frame 53 {
          n117 = call "WILT Cutout Delay.vi"("Delay After Cutout (sec)"=w458, "Cut-In?"=TRUE, "Error In"=w461, "Current Threshold"=w462, "L2 Current"=w463, "L1 Current"=w464) -> ("Error Out"=w460:errorcluster, "Delayed Trigger"=w459:bool)  [unwired: 2 in, 2 out]
        }
        frame 54 {
          n118 = call "WILT Cutout Delay.vi"("Delay After Cutout (sec)"=w466, "Cut-In?"=TRUE, "Error In"=w469, "Current Threshold"=w470, "L2 Current"=w471, "L1 Current"=w472) -> ("Error Out"=w468:errorcluster, "Delayed Trigger"=w467:bool)  [unwired: 2 in, 2 out]
        }
        frame 55 {
          n119 = call "WILT Cutout Delay.vi"("Delay After Cutout (sec)"=w474, "Cut-In?"=TRUE, "Error In"=w477, "Current Threshold"=w478, "L2 Current"=w479, "L1 Current"=w480) -> ("Error Out"=w476:errorcluster, "Delayed Trigger"=w475:bool)  [unwired: 2 in, 2 out]
        }
        frame 56 {
          n120 = call "WILT Cutout Delay.vi"("Delay After Cutout (sec)"=w484, "Cut-In?"=TRUE, "Error In"=w485, "Current Threshold"=w486, "L2 Current"=w487, "L1 Current"=w488) -> ("Error Out"=w483:errorcluster, "Delayed Trigger"=w482:bool)  [unwired: 2 in, 2 out]
        }
      }
      n121 = Equal?(x=w32, y=w33) -> (x = y?=w31:bool)
      n122 = case shown="True" w31 {
        tunnel: [FALSE TRUE] -> w30
        frame False {
        }
        frame True {
        }
      }
      n123 = Compound Arithmetic op=AND(invert w22, "Enable Start Retry") -> (w21:bool)
      n124 = case shown="6" w13 {
        tunnel: [w497 w498 w500 w502 w504 w506 w508 w510 w512 w514 w516 w518 w520 w522 w524 w526 w528 w530 w532 w534 w536 w538 w540 w542 w544 w546 w548 w550 w552 w554 w556 w558 w560 w562 w564 w566 w568 w570 w572 w574 w576 w578 w580 w582 w584 w586 w588 w590 w592 w594 w596 w598 w600 w602 w604 w606] -> w28
        tunnel: w30 -> [w496 w499 w501 w503 w505 w507 w509 w511 w513 w515 w517 w519 w521 w523 w525 w527 w529 w531 w533 w535 w537 w539 w541 w543 w545 w547 w549 w551 w553 w555 w557 w559 w561 w563 w565 w567 w569 w571 w573 w575 w577 w579 w581 w583 w585 w587 w589 w591 w593 w595 w597 w599 w601 w603 w605 w607]
        frame 1, Default {
          n125 = call "UTILITY E-Time.vi"("Reset"=w496) -> ("Elapsed Time (sec)"=w497:dbl)  [unwired: 8 in, 2 out]
        }
        frame 2 {
          n126 = call "UTILITY E-Time.vi"("Reset"=w499) -> ("Elapsed Time (sec)"=w498:dbl)  [unwired: 8 in, 2 out]
        }
        frame 3 {
          n127 = call "UTILITY E-Time.vi"("Reset"=w501) -> ("Elapsed Time (sec)"=w500:dbl)  [unwired: 8 in, 2 out]
        }
        frame 4 {
          n128 = call "UTILITY E-Time.vi"("Reset"=w503) -> ("Elapsed Time (sec)"=w502:dbl)  [unwired: 8 in, 2 out]
        }
        frame 5 {
          n129 = call "UTILITY E-Time.vi"("Reset"=w505) -> ("Elapsed Time (sec)"=w504:dbl)  [unwired: 8 in, 2 out]
        }
        frame 6 {
          n130 = call "UTILITY E-Time.vi"("Reset"=w507) -> ("Elapsed Time (sec)"=w506:dbl)  [unwired: 8 in, 2 out]
        }
        frame 7 {
          n131 = call "UTILITY E-Time.vi"("Reset"=w509) -> ("Elapsed Time (sec)"=w508:dbl)  [unwired: 8 in, 2 out]
        }
        frame 8 {
          n132 = call "UTILITY E-Time.vi"("Reset"=w511) -> ("Elapsed Time (sec)"=w510:dbl)  [unwired: 8 in, 2 out]
        }
        frame 9 {
          n133 = call "UTILITY E-Time.vi"("Reset"=w513) -> ("Elapsed Time (sec)"=w512:dbl)  [unwired: 8 in, 2 out]
        }
        frame 10 {
          n134 = call "UTILITY E-Time.vi"("Reset"=w515) -> ("Elapsed Time (sec)"=w514:dbl)  [unwired: 8 in, 2 out]
        }
        frame 11 {
          n135 = call "UTILITY E-Time.vi"("Reset"=w517) -> ("Elapsed Time (sec)"=w516:dbl)  [unwired: 8 in, 2 out]
        }
        frame 12 {
          n136 = call "UTILITY E-Time.vi"("Reset"=w519) -> ("Elapsed Time (sec)"=w518:dbl)  [unwired: 8 in, 2 out]
        }
        frame 13 {
          n137 = call "UTILITY E-Time.vi"("Reset"=w521) -> ("Elapsed Time (sec)"=w520:dbl)  [unwired: 8 in, 2 out]
        }
        frame 14 {
          n138 = call "UTILITY E-Time.vi"("Reset"=w523) -> ("Elapsed Time (sec)"=w522:dbl)  [unwired: 8 in, 2 out]
        }
        frame 15 {
          n139 = call "UTILITY E-Time.vi"("Reset"=w525) -> ("Elapsed Time (sec)"=w524:dbl)  [unwired: 8 in, 2 out]
        }
        frame 16 {
          n140 = call "UTILITY E-Time.vi"("Reset"=w527) -> ("Elapsed Time (sec)"=w526:dbl)  [unwired: 8 in, 2 out]
        }
        frame 17 {
          n141 = call "UTILITY E-Time.vi"("Reset"=w529) -> ("Elapsed Time (sec)"=w528:dbl)  [unwired: 8 in, 2 out]
        }
        frame 18 {
          n142 = call "UTILITY E-Time.vi"("Reset"=w531) -> ("Elapsed Time (sec)"=w530:dbl)  [unwired: 8 in, 2 out]
        }
        frame 19 {
          n143 = call "UTILITY E-Time.vi"("Reset"=w533) -> ("Elapsed Time (sec)"=w532:dbl)  [unwired: 8 in, 2 out]
        }
        frame 20 {
          n144 = call "UTILITY E-Time.vi"("Reset"=w535) -> ("Elapsed Time (sec)"=w534:dbl)  [unwired: 8 in, 2 out]
        }
        frame 21 {
          n145 = call "UTILITY E-Time.vi"("Reset"=w537) -> ("Elapsed Time (sec)"=w536:dbl)  [unwired: 8 in, 2 out]
        }
        frame 22 {
          n146 = call "UTILITY E-Time.vi"("Reset"=w539) -> ("Elapsed Time (sec)"=w538:dbl)  [unwired: 8 in, 2 out]
        }
        frame 23 {
          n147 = call "UTILITY E-Time.vi"("Reset"=w541) -> ("Elapsed Time (sec)"=w540:dbl)  [unwired: 8 in, 2 out]
        }
        frame 24 {
          n148 = call "UTILITY E-Time.vi"("Reset"=w543) -> ("Elapsed Time (sec)"=w542:dbl)  [unwired: 8 in, 2 out]
        }
        frame 25 {
          n149 = call "UTILITY E-Time.vi"("Reset"=w545) -> ("Elapsed Time (sec)"=w544:dbl)  [unwired: 8 in, 2 out]
        }
        frame 26 {
          n150 = call "UTILITY E-Time.vi"("Reset"=w547) -> ("Elapsed Time (sec)"=w546:dbl)  [unwired: 8 in, 2 out]
        }
        frame 27 {
          n151 = call "UTILITY E-Time.vi"("Reset"=w549) -> ("Elapsed Time (sec)"=w548:dbl)  [unwired: 8 in, 2 out]
        }
        frame 28 {
          n152 = call "UTILITY E-Time.vi"("Reset"=w551) -> ("Elapsed Time (sec)"=w550:dbl)  [unwired: 8 in, 2 out]
        }
        frame 29 {
          n153 = call "UTILITY E-Time.vi"("Reset"=w553) -> ("Elapsed Time (sec)"=w552:dbl)  [unwired: 8 in, 2 out]
        }
        frame 30 {
          n154 = call "UTILITY E-Time.vi"("Reset"=w555) -> ("Elapsed Time (sec)"=w554:dbl)  [unwired: 8 in, 2 out]
        }
        frame 31 {
          n155 = call "UTILITY E-Time.vi"("Reset"=w557) -> ("Elapsed Time (sec)"=w556:dbl)  [unwired: 8 in, 2 out]
        }
        frame 32 {
          n156 = call "UTILITY E-Time.vi"("Reset"=w559) -> ("Elapsed Time (sec)"=w558:dbl)  [unwired: 8 in, 2 out]
        }
        frame 33 {
          n157 = call "UTILITY E-Time.vi"("Reset"=w561) -> ("Elapsed Time (sec)"=w560:dbl)  [unwired: 8 in, 2 out]
        }
        frame 34 {
          n158 = call "UTILITY E-Time.vi"("Reset"=w563) -> ("Elapsed Time (sec)"=w562:dbl)  [unwired: 8 in, 2 out]
        }
        frame 35 {
          n159 = call "UTILITY E-Time.vi"("Reset"=w565) -> ("Elapsed Time (sec)"=w564:dbl)  [unwired: 8 in, 2 out]
        }
        frame 36 {
          n160 = call "UTILITY E-Time.vi"("Reset"=w567) -> ("Elapsed Time (sec)"=w566:dbl)  [unwired: 8 in, 2 out]
        }
        frame 37 {
          n161 = call "UTILITY E-Time.vi"("Reset"=w569) -> ("Elapsed Time (sec)"=w568:dbl)  [unwired: 8 in, 2 out]
        }
        frame 38 {
          n162 = call "UTILITY E-Time.vi"("Reset"=w571) -> ("Elapsed Time (sec)"=w570:dbl)  [unwired: 8 in, 2 out]
        }
        frame 39 {
          n163 = call "UTILITY E-Time.vi"("Reset"=w573) -> ("Elapsed Time (sec)"=w572:dbl)  [unwired: 8 in, 2 out]
        }
        frame 40 {
          n164 = call "UTILITY E-Time.vi"("Reset"=w575) -> ("Elapsed Time (sec)"=w574:dbl)  [unwired: 8 in, 2 out]
        }
        frame 41 {
          n165 = call "UTILITY E-Time.vi"("Reset"=w577) -> ("Elapsed Time (sec)"=w576:dbl)  [unwired: 8 in, 2 out]
        }
        frame 42 {
          n166 = call "UTILITY E-Time.vi"("Reset"=w579) -> ("Elapsed Time (sec)"=w578:dbl)  [unwired: 8 in, 2 out]
        }
        frame 43 {
          n167 = call "UTILITY E-Time.vi"("Reset"=w581) -> ("Elapsed Time (sec)"=w580:dbl)  [unwired: 8 in, 2 out]
        }
        frame 44 {
          n168 = call "UTILITY E-Time.vi"("Reset"=w583) -> ("Elapsed Time (sec)"=w582:dbl)  [unwired: 8 in, 2 out]
        }
        frame 45 {
          n169 = call "UTILITY E-Time.vi"("Reset"=w585) -> ("Elapsed Time (sec)"=w584:dbl)  [unwired: 8 in, 2 out]
        }
        frame 46 {
          n170 = call "UTILITY E-Time.vi"("Reset"=w587) -> ("Elapsed Time (sec)"=w586:dbl)  [unwired: 8 in, 2 out]
        }
        frame 47 {
          n171 = call "UTILITY E-Time.vi"("Reset"=w589) -> ("Elapsed Time (sec)"=w588:dbl)  [unwired: 8 in, 2 out]
        }
        frame 48 {
          n172 = call "UTILITY E-Time.vi"("Reset"=w591) -> ("Elapsed Time (sec)"=w590:dbl)  [unwired: 8 in, 2 out]
        }
        frame 49 {
          n173 = call "UTILITY E-Time.vi"("Reset"=w593) -> ("Elapsed Time (sec)"=w592:dbl)  [unwired: 8 in, 2 out]
        }
        frame 50 {
          n174 = call "UTILITY E-Time.vi"("Reset"=w595) -> ("Elapsed Time (sec)"=w594:dbl)  [unwired: 8 in, 2 out]
        }
        frame 51 {
          n175 = call "UTILITY E-Time.vi"("Reset"=w597) -> ("Elapsed Time (sec)"=w596:dbl)  [unwired: 8 in, 2 out]
        }
        frame 52 {
          n176 = call "UTILITY E-Time.vi"("Reset"=w599) -> ("Elapsed Time (sec)"=w598:dbl)  [unwired: 8 in, 2 out]
        }
        frame 53 {
          n177 = call "UTILITY E-Time.vi"("Reset"=w601) -> ("Elapsed Time (sec)"=w600:dbl)  [unwired: 8 in, 2 out]
        }
        frame 54 {
          n178 = call "UTILITY E-Time.vi"("Reset"=w603) -> ("Elapsed Time (sec)"=w602:dbl)  [unwired: 8 in, 2 out]
        }
        frame 55 {
          n179 = call "UTILITY E-Time.vi"("Reset"=w605) -> ("Elapsed Time (sec)"=w604:dbl)  [unwired: 8 in, 2 out]
        }
        frame 56 {
          n180 = call "UTILITY E-Time.vi"("Reset"=w607) -> ("Elapsed Time (sec)"=w606:dbl)  [unwired: 8 in, 2 out]
        }
      }
      n181 = Select(t=WILT_Dryer_Test_State."Drying Clothes" ("Station Test State Input 2"), s=w17, f=w34) -> (s? t:f=w36:T3)
      n182 = case shown="False" w21 {
        tunnel: w28 -> [_ w493]
        tunnel: w27 -> [_ w491]
        tunnel: w13 -> [_ w490]
        frame False {
        }
        frame True {
          n183 = call "WILT Interval Resend.vi"("Send Restart Every? (Sec)"="Send Restart Every? (Sec)", "Elapsed Time (sec)"=w493, "Station Number in"=w490, "Agilent Valve and Switch Locations"=w491) -> ("Sending CMD"=→"Resending Sending Command":bool)  [unwired: 7 in]
        }
      }
      n184 = case shown="1" w13 {
        tunnel: w35 -> [w721 w724 w727 w730 w733 w736 w739 w742 w745 w748 w751 w754 w757 w760 w763 w766 w769 w772 w775 w778 w781 w784 w787 w790 w793 w796 w799 w802 w805 w808 w811 w814 w817 w820 w823 w826 w829 w832 w835 w838 w841 w844 w847 w850 w853 w856 w859 w862 w865 w868 w871 w874 w877 w880 w883 w886 w889]
        tunnel: w36 -> [_ w723 w725 w728 w731 w734 w737 w740 w743 w746 w749 w752 w755 w758 w761 w764 w767 w770 w773 w776 w779 w782 w785 w788 w791 w794 w797 w800 w803 w806 w809 w812 w815 w818 w821 w824 w827 w830 w833 w836 w839 w842 w845 w848 w851 w854 w857 w860 w863 w866 w869 w872 w875 w878 w881 w884 w887]
        tunnel: [w721 w722 w726 w729 w732 w735 w738 w741 w744 w747 w750 w753 w756 w759 w762 w765 w768 w771 w774 w777 w780 w783 w786 w789 w792 w795 w798 w801 w804 w807 w810 w813 w816 w819 w822 w825 w828 w831 w834 w837 w840 w843 w846 w849 w852 w855 w858 w861 w864 w867 w870 w873 w876 w879 w882 w885 w888] -> w38
        frame 0, Default {
          # "Not a valid station. Do nothing"
        }
        frame 1 {
          n185 = Bundle By Name(cluster=w724, "Station Test State 1"=w723) -> (w722:T2)
        }
        frame 2 {
          n186 = Bundle By Name(cluster=w727, "Station Test State 2"=w725) -> (w726:T2)
        }
        frame 3 {
          n187 = Bundle By Name(cluster=w730, "Station Test State 3"=w728) -> (w729:T2)
        }
        frame 4 {
          n188 = Bundle By Name(cluster=w733, "Station Test State 4"=w731) -> (w732:T2)
        }
        frame 5 {
          n189 = Bundle By Name(cluster=w736, "Station Test State 5"=w734) -> (w735:T2)
        }
        frame 6 {
          n190 = Bundle By Name(cluster=w739, "Station Test State 6"=w737) -> (w738:T2)
        }
        frame 7 {
          n191 = Bundle By Name(cluster=w742, "Station Test State 7"=w740) -> (w741:T2)
        }
        frame 8 {
          n192 = Bundle By Name(cluster=w745, "Station Test State 8"=w743) -> (w744:T2)
        }
        frame 9 {
          n193 = Bundle By Name(cluster=w748, "Station Test State 9"=w746) -> (w747:T2)
        }
        frame 10 {
          n194 = Bundle By Name(cluster=w751, "Station Test State 10"=w749) -> (w750:T2)
        }
        frame 11 {
          n195 = Bundle By Name(cluster=w754, "Station Test State 11"=w752) -> (w753:T2)
        }
        frame 12 {
          n196 = Bundle By Name(cluster=w757, "Station Test State 12"=w755) -> (w756:T2)
        }
        frame 13 {
          n197 = Bundle By Name(cluster=w760, "Station Test State 13"=w758) -> (w759:T2)
        }
        frame 14 {
          n198 = Bundle By Name(cluster=w763, "Station Test State 14"=w761) -> (w762:T2)
        }
        frame 15 {
          n199 = Bundle By Name(cluster=w766, "Station Test State 15"=w764) -> (w765:T2)
        }
        frame 16 {
          n200 = Bundle By Name(cluster=w769, "Station Test State 16"=w767) -> (w768:T2)
        }
        frame 17 {
          n201 = Bundle By Name(cluster=w772, "Station Test State 17"=w770) -> (w771:T2)
        }
        frame 18 {
          n202 = Bundle By Name(cluster=w775, "Station Test State 18"=w773) -> (w774:T2)
        }
        frame 19 {
          n203 = Bundle By Name(cluster=w778, "Station Test State 19"=w776) -> (w777:T2)
        }
        frame 20 {
          n204 = Bundle By Name(cluster=w781, "Station Test State 20"=w779) -> (w780:T2)
        }
        frame 21 {
          n205 = Bundle By Name(cluster=w784, "Station Test State 21"=w782) -> (w783:T2)
        }
        frame 22 {
          n206 = Bundle By Name(cluster=w787, "Station Test State 22"=w785) -> (w786:T2)
        }
        frame 23 {
          n207 = Bundle By Name(cluster=w790, "Station Test State 23"=w788) -> (w789:T2)
        }
        frame 24 {
          n208 = Bundle By Name(cluster=w793, "Station Test State 24"=w791) -> (w792:T2)
        }
        frame 25 {
          n209 = Bundle By Name(cluster=w796, "Station Test State 25"=w794) -> (w795:T2)
        }
        frame 26 {
          n210 = Bundle By Name(cluster=w799, "Station Test State 26"=w797) -> (w798:T2)
        }
        frame 27 {
          n211 = Bundle By Name(cluster=w802, "Station Test State 27"=w800) -> (w801:T2)
        }
        frame 28 {
          n212 = Bundle By Name(cluster=w805, "Station Test State 28"=w803) -> (w804:T2)
        }
        frame 29 {
          n213 = Bundle By Name(cluster=w808, "Station Test State 29"=w806) -> (w807:T2)
        }
        frame 30 {
          n214 = Bundle By Name(cluster=w811, "Station Test State 30"=w809) -> (w810:T2)
        }
        frame 31 {
          n215 = Bundle By Name(cluster=w814, "Station Test State 31"=w812) -> (w813:T2)
        }
        frame 32 {
          n216 = Bundle By Name(cluster=w817, "Station Test State 32"=w815) -> (w816:T2)
        }
        frame 33 {
          n217 = Bundle By Name(cluster=w820, "Station Test State 33"=w818) -> (w819:T2)
        }
        frame 34 {
          n218 = Bundle By Name(cluster=w823, "Station Test State 34"=w821) -> (w822:T2)
        }
        frame 35 {
          n219 = Bundle By Name(cluster=w826, "Station Test State 35"=w824) -> (w825:T2)
        }
        frame 36 {
          n220 = Bundle By Name(cluster=w829, "Station Test State 36"=w827) -> (w828:T2)
        }
        frame 37 {
          n221 = Bundle By Name(cluster=w832, "Station Test State 37"=w830) -> (w831:T2)
        }
        frame 38 {
          n222 = Bundle By Name(cluster=w835, "Station Test State 38"=w833) -> (w834:T2)
        }
        frame 39 {
          n223 = Bundle By Name(cluster=w838, "Station Test State 39"=w836) -> (w837:T2)
        }
        frame 40 {
          n224 = Bundle By Name(cluster=w841, "Station Test State 40"=w839) -> (w840:T2)
        }
        frame 41 {
          n225 = Bundle By Name(cluster=w844, "Station Test State 41"=w842) -> (w843:T2)
        }
        frame 42 {
          n226 = Bundle By Name(cluster=w847, "Station Test State 42"=w845) -> (w846:T2)
        }
        frame 43 {
          n227 = Bundle By Name(cluster=w850, "Station Test State 43"=w848) -> (w849:T2)
        }
        frame 44 {
          n228 = Bundle By Name(cluster=w853, "Station Test State 44"=w851) -> (w852:T2)
        }
        frame 45 {
          n229 = Bundle By Name(cluster=w856, "Station Test State 45"=w854) -> (w855:T2)
        }
        frame 46 {
          n230 = Bundle By Name(cluster=w859, "Station Test State 46"=w857) -> (w858:T2)
        }
        frame 47 {
          n231 = Bundle By Name(cluster=w862, "Station Test State 47"=w860) -> (w861:T2)
        }
        frame 48 {
          n232 = Bundle By Name(cluster=w865, "Station Test State 48"=w863) -> (w864:T2)
        }
        frame 49 {
          n233 = Bundle By Name(cluster=w868, "Station Test State 49"=w866) -> (w867:T2)
        }
        frame 50 {
          n234 = Bundle By Name(cluster=w871, "Station Test State 50"=w869) -> (w870:T2)
        }
        frame 51 {
          n235 = Bundle By Name(cluster=w874, "Station Test State 51"=w872) -> (w873:T2)
        }
        frame 52 {
          n236 = Bundle By Name(cluster=w877, "Station Test State 52"=w875) -> (w876:T2)
        }
        frame 53 {
          n237 = Bundle By Name(cluster=w880, "Station Test State 53"=w878) -> (w879:T2)
        }
        frame 54 {
          n238 = Bundle By Name(cluster=w883, "Station Test State 54"=w881) -> (w882:T2)
        }
        frame 55 {
          n239 = Bundle By Name(cluster=w886, "Station Test State 55"=w884) -> (w885:T2)
        }
        frame 56 {
          n240 = Bundle By Name(cluster=w889, "Station Test State 56"=w887) -> (w888:T2)
        }
      }
    }
    frame #1 {
      n241 = global read "WILT Globals Main Program.vi" "EOC"() -> (w892:u32)
      n242 = Bundle By Name(cluster=w890, "Status Color"=w892) -> (w891:T4)
    }
  }
  "Dryer Output" <- w7
  "Error Out" <- w3
  "Step 2 Output" <- w12
